vi "Interface-IF2004_USB.vi"() -> ()   [LabVIEW 2015, in "MEDAQLib.lvlib"]
uses:
  MEDAQLib.lvlib
panel:
  out "Last error text":string
  in  "Channel":i32 min=0 max=3
  in  "COM Port":string="COM3"
  in  "Sensor type":string="ifd2451"
  out "ScaledData":dbl[](graph)
  in  "stop":bool
  in  "Block size":i32=200
  # "1. Preparations\nPlease use Sensor tool to find sensor connected to your PC and get its interface/communication parameters."
  # "2. Inform MEDAQLib about sensor type and interface parameters.\nFor possible sensor type names see MEDAQLib.h or CreateSensorInstByName documentation in MEDAQLib.pdf\nCOM Port = Port of IF2004_USB\nChannel = Channel at IF2004_USB, where your sensor is connected to (0..3)\n\nPlease note: this example expects to access the sensor with its default baudrate. You may need to insert another SetParameterInt VI to tell MEDAQLib about a changed baudrate."
  # "3. Start LabView execution"
  # "4. For stop please do not use LabView red stop button on toolbar, but the red STOP button below to be able to inform MEDAQLib about release of sensor instance information."
  # "Number of samples\nper transfered data block"
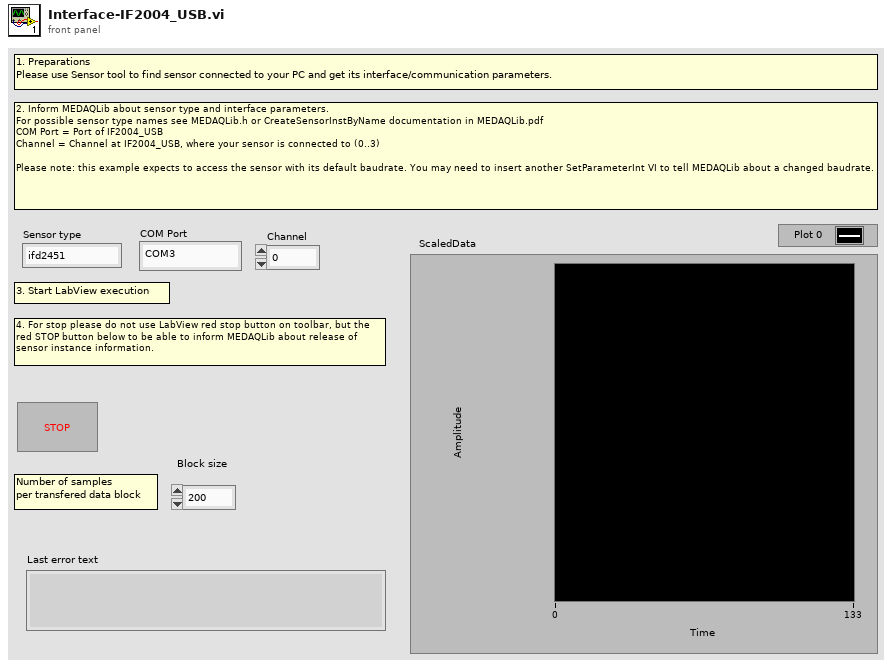
[diagram p1: front panel]
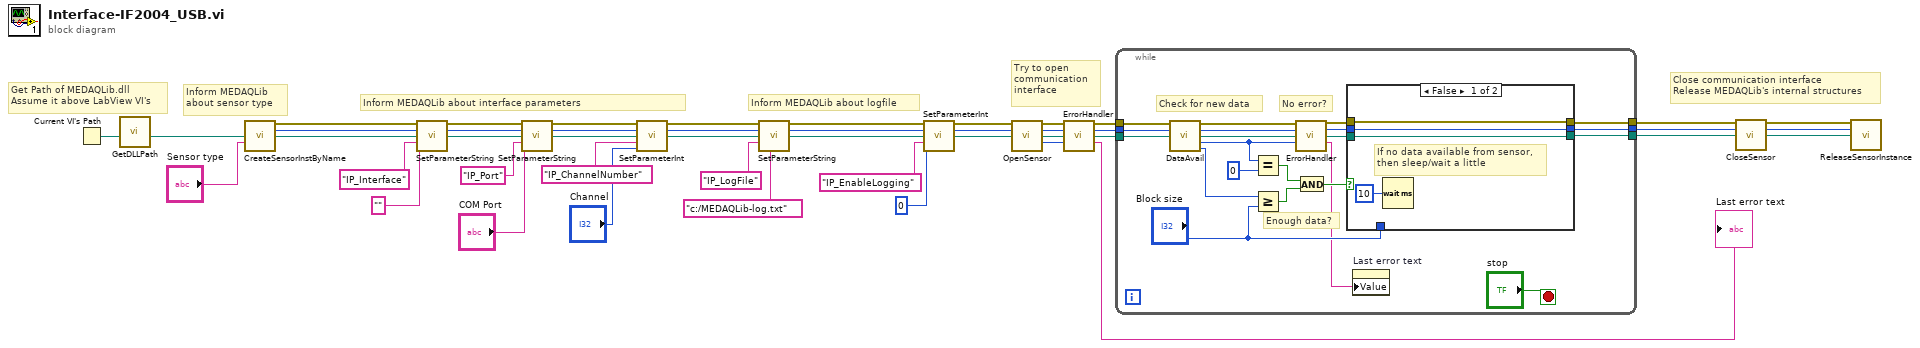
[diagram p0: block diagram]
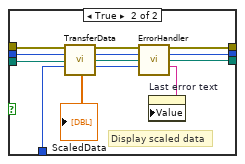
[diagram p2: hidden frame]
diagram:
  # "Close communication interface\nRelease MEDAQLib's internal structures"
  # "Try to open\ncommunication\ninterface"
  # "Inform MEDAQLib about logfile"
  # "Inform MEDAQLib about interface parameters"
  # "Inform MEDAQLib\nabout sensor type"
  # "Get Path of MEDAQLib.dll\nAssume it above LabView VI's"
  n1 = Current VI's Path() -> (path=w17:path)
  n2 = call "GetDLLPath.vi"("VI-Path"=w17) -> ("DLL-Path"=w18:path)  [unwired: 10 out]
  n3 = call "CreateSensorInstByName.vi"("DLL-Path"=w18, "sensor"="Sensor type") -> ("Fehler (Ausgang)"=w44:errorcluster, "instanceHandle"=w43:u32, "DLL-Path"=w42:path)  [unwired: 1 in, 10 out]
  n4 = call "SetParameterString.vi"("Fehler (Eingang, kein Fehler)"=w44, "instanceHandle"=w43, "DLL-Path"=w42, "paramName"="IP_Interface", "paramValue"="") -> ("Fehler (Ausgang)"=w39:errorcluster, "instanceHandle"=w38:u32, "DLL-Path"=w37:path)  [unwired: 8 out]
  n5 = call "SetParameterString.vi"("Fehler (Eingang, kein Fehler)"=w39, "instanceHandle"=w38, "DLL-Path"=w37, "paramName"="IP_Port", "paramValue"="COM Port") -> ("Fehler (Ausgang)"=w16:errorcluster, "instanceHandle"=w15:u32, "DLL-Path"=w12:path)  [unwired: 8 out]
  n6 = call "SetParameterInt.vi"("Fehler (Eingang, kein Fehler)"=w16, "instanceHandle"=w15, "DLL-Path"=w12, "paramName"="IP_ChannelNumber", "paramValue"="Channel") -> ("Fehler (Ausgang)"=w14:errorcluster, "instanceHandle"=w13:u32, "DLL-Path"=w11:path)  [unwired: 8 out]
  n7 = call "SetParameterString.vi"("Fehler (Eingang, kein Fehler)"=w14, "instanceHandle"=w13, "DLL-Path"=w11, "paramName"="IP_LogFile", "paramValue"="c:/MEDAQLib-log.txt") -> ("Fehler (Ausgang)"=w32:errorcluster, "instanceHandle"=w31:u32, "DLL-Path"=w30:path)  [unwired: 8 out]
  n8 = call "SetParameterInt.vi"("Fehler (Eingang, kein Fehler)"=w32, "instanceHandle"=w31, "DLL-Path"=w30, "paramName"="IP_EnableLogging", "paramValue"=0) -> ("Fehler (Ausgang)"=w27:errorcluster, "instanceHandle"=w26:u32, "DLL-Path"=w25:path)  [unwired: 8 out]
  n9 = call "OpenSensor.vi"("Fehler (Eingang, kein Fehler)"=w27, "instanceHandle"=w26, "DLL-Path"=w25) -> ("Fehler (Ausgang)"=w8:errorcluster, "instanceHandle"=w7:u32, "DLL-Path"=w6:path, "ERR_CODE"=w5:i32)  [unwired: 1 in, 8 out]
  n10 = call "ErrorHandler.vi"("Fehler (Eingang, kein Fehler)"=w8, "instanceHandle"=w7, "DLL-Path"=w6, "ERR_CODE"=w5) -> ("Fehler (Ausgang)"=w4:errorcluster, "instanceHandle"=w3:u32, "DLL-Path"=w2:path, "errText"=→"Last error text":string)  [unwired: 8 out]
  n11 = while {
    tunnel: w4 -> [w66]
    tunnel: w3 -> [w65]
    tunnel: w2 -> [w64]
    tunnel: [w59] -> w24
    tunnel: [w58] -> w23
    tunnel: [w57] -> w22
    stop <- "stop" stop-if-true
    # "Enough data?"
    # "No error?"
    # "Check for new data"
    n12 = call "DataAvail.vi"("Fehler (Eingang, kein Fehler)"=w66, "instanceHandle"=w65, "DLL-Path"=w64) -> ("Fehler (Ausgang)"=w53:errorcluster, "instanceHandle"=w51:u32, "DLL-Path"=w49:path, "ERR_CODE"=w47:i32, "avail"=w63:i32)  [unwired: 8 out]
    n13 = Equal?(x=w47, y=0 ("x")) -> (x = y?=w60:bool)
    n14 = Greater Or Equal?(x=w63, y="Block size") -> (x >= y?=w56:bool)
    n15 = call "ErrorHandler.vi"("Fehler (Eingang, kein Fehler)"=w53, "instanceHandle"=w51, "DLL-Path"=w49, "ERR_CODE"=w47) -> ("Fehler (Ausgang)"=w52:errorcluster, "instanceHandle"=w50:u32, "DLL-Path"=w48:path, "errText"=w46:string)  [unwired: 8 out]
    n16 = And(x=w60, y=w56) -> (x .and. y?=w61:bool)
    n17 = case shown="False" w61 {
      tunnel: w52 -> [w70 w82]
      tunnel: w50 -> [w69 w83]
      tunnel: w48 -> [w68 w81]
      tunnel: [w70 w77] -> w59
      tunnel: [w69 w75] -> w58
      tunnel: [w68 w73] -> w57
      tunnel: "Block size" -> [_ w80]
      frame False {
        # "If no data available from sensor,\nthen sleep/wait a little"
        n18 = Wait (ms)(milliseconds to wait=u32 10 ("Zu wartende ms")) -> ()  [unwired: 1 out]
      }
      frame True {
        # "Display scaled data"
        n19 = call "TransferData.vi"("Fehler (Eingang, kein Fehler)"=w82, "instanceHandle"=w83, "DLL-Path"=w81, "maxValues"=w80) -> ("Fehler (Ausgang)"=w78:errorcluster, "instanceHandle"=w76:u32, "DLL-Path"=w74:path, "ERR_CODE"=w71:i32, "scaledData"=→"ScaledData":dbl[])  [unwired: 7 out]
        n20 = call "ErrorHandler.vi"("Fehler (Eingang, kein Fehler)"=w78, "instanceHandle"=w76, "DLL-Path"=w74, "ERR_CODE"=w71) -> ("Fehler (Ausgang)"=w77:errorcluster, "instanceHandle"=w75:u32, "DLL-Path"=w73:path, "errText"=w72:string)  [unwired: 8 out]
        n21 = property on="Last error text" class="Str"("Value"=w72) -> ()  [unwired: 2 in, 2 out]
      }
    }
    n22 = property on="Last error text" class="Str"("Value"=w46) -> ()  [unwired: 2 in, 2 out]
  }
  n23 = call "CloseSensor.vi"("Fehler (Eingang, kein Fehler)"=w24, "instanceHandle"=w23, "DLL-Path"=w22) -> ("Fehler (Ausgang)"=w21:errorcluster, "instanceHandle"=w20:u32, "DLL-Path"=w19:path)  [unwired: 10 out]
  n24 = call "ReleaseSensorInstance.vi"("Fehler (Eingang, kein Fehler)"=w21, "instanceHandle"=w20, "DLL-Path"=w19) -> ()  [unwired: 13 out]
